vi "Real SVD Decomposition.vi"(9 "SVD option":T2 items=["Thin", "Full"], 10 "singular values only?":bool, 11 "A":T1) -> (0 "error":i32, 1 "Matrix V":T1, 2 "Matrix S":T1, 3 "Matrix U":T1, 5 "Vector S":dbl[](array[numeric]))   [LabVIEW 2010, in "NI_AALPro.lvlib"]
doc: "Computes the singular value decomposition (SVD) of the m x n matrix <B>A</B>. Wire data to the <B>A</B> input to determine the polymorphic instance to use or manually select the instance."
uses:
  NI_AALPro.lvlib
  RealMatrix.ctl
  SVD Option.ctl
  Create Special Real Matrix.vi
  lvanlys.dll
  NI_Matrix.lvlib
panel:
  # "SVD Decomposition"
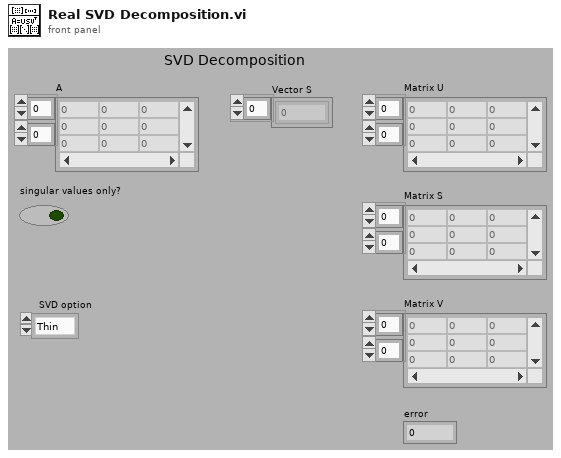
[diagram p1: front panel]
types:
  T1 = typedef "NI_Matrix.lvlib/RealMatrix.ctl" = dbl[][]
  T2 = typedef "NI_AALPro.lvlib/SVD Option.ctl" = u16
  T3 = enum32{"Identity", "Diagonal", "Toepliz", "Vandermonde", "Companion"}
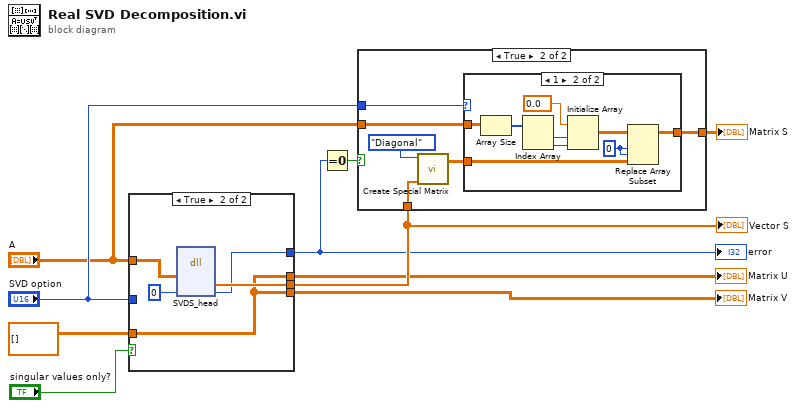
[diagram p0: block diagram]
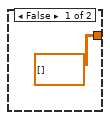
[diagram p2: hidden frame]
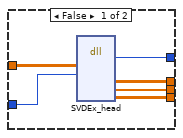
[diagram p4: hidden frame]
diagram:
  n1 = case shown="True" "singular values only?" {
    tunnel: [w13 w17] -> w5
    tunnel: [w16 w18] -> w2
    tunnel: "SVD option" -> [w15 _]
    tunnel: [w12 w19] -> w9
    tunnel: "A" -> [w14 w21]
    tunnel: [w11 w17] -> w6
    tunnel: dbl[][] [] ("V") -> [_ w17]
    frame False {
      n2 = dll-call lib="C:/Program Files/National Instruments/LabVIEW 2010/resource/lvanlys.*" fn="SVDEx_head"("aH"=w14, "flag"=w15) -> ("return type"=w16:i32, "uH"=w13:dbl[][], "sH"=w12:dbl[], "vH"=w11:dbl[][])  [unwired: 8 in, 2 out]
    }
    frame True {
      n3 = dll-call lib="C:/Program Files/National Instruments/LabVIEW 2010/resource/lvanlys.*" fn="SVDS_head"("aH"=w21, "dsperr"=0 ("input param")) -> ("wH"=w19:dbl[], "dsperr"=w18:i32)  [unwired: 6 in, 2 out]
    }
  }
  "Matrix U" <- w5
  "Matrix V" <- w6
  "error" <- w2
  "Vector S" <- w9
  n4 = Equal To 0?(x=w2) -> (x = 0?=w3:bool)
  n5 = case shown="True" w3 {
    tunnel: "SVD option" -> [_ w28]
    tunnel: w9 -> [_ w27]
    tunnel: "A" -> [_ w24]
    tunnel: [dbl[][] [] ("Special Matrix") w23] -> w4
    frame False {
    }
    frame True {
      n6 = call-poly "Create Special Matrix.vi"("matrix type"=T3."Diagonal", "Input Vector1"=w27) -> ("Special Matrix"=w25:T1)  [unwired: 3 in, 1 out]
      n7 = case shown="1" w28 {
        tunnel: [w29 w30] -> w23
        tunnel: w25 -> [w29 w31]
        tunnel: w24 -> [_ w35]
        frame 0, Default {
        }
        frame 1 {
          w32 = 0 ("index (row)")
          n8 = Array Size(array=w35) -> (size(s)=w34:i32[])
          n9 = Index Array(array=w34) -> (element #1=w37:i32, element #2=w36:i32)  [unwired: 2 in]
          n10 = Initialize Array(0.0 ("element"), w37, w36) -> (w33:dbl[][])
          n11 = Replace Array Subset(array=w33, new element=w31, index (row)=w32, index (col)=w32) -> (w30:dbl[][])
        }
      }
    }
  }
  "Matrix S" <- w4
